vi "Priority.vi"(8 "error in (no error)":errorcluster, 11 "Request Session Handler in":refnum<class "Request Session Handler.lvclass">) -> (0 "error out":errorcluster, 2 "Priority":u16, 3 "Request Session Handler out":refnum<class "Request Session Handler.lvclass">)   [LabVIEW 2020, in "HTTP Server.lvlib" / "Request Session Handler.lvclass"]
uses:
  Request Session Handler.lvclass
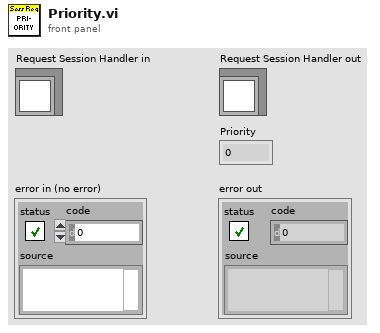
[diagram p1: front panel]
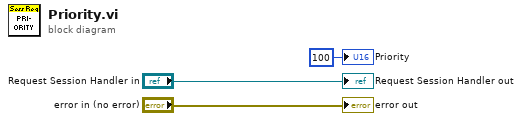
[diagram p0: block diagram]
diagram:
  "error out" <- "error in (no error)"
  "Request Session Handler out" <- "Request Session Handler in"
  "Priority" <- u16 100 ("Priority")
